vi "Filter Traces.vi"(8 "error in (no error)":errorcluster, 9 "Median Filter?":bool, 10 "Array":cluster{timestamp[], dbl[]}[](array[cluster]), 11 "Database Viewer in":refnum<class "Database Viewer.lvclass">) -> (0 "error out":errorcluster, 2 "Database Trace out":T1(array[cluster]), 3 "Database Viewer out":refnum<class "Database Viewer.lvclass">)   [LabVIEW 2019, in "Database Viewer.lvclass"]
uses:
  Database Viewer.lvclass
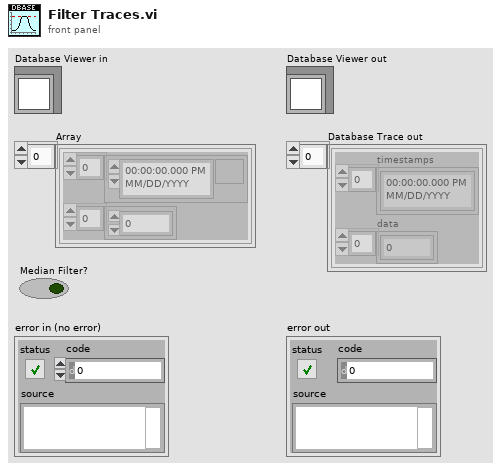
[diagram p1: front panel]
types:
  T1 = cluster{"timestamps":timestamp[], "data":dbl[]}[]
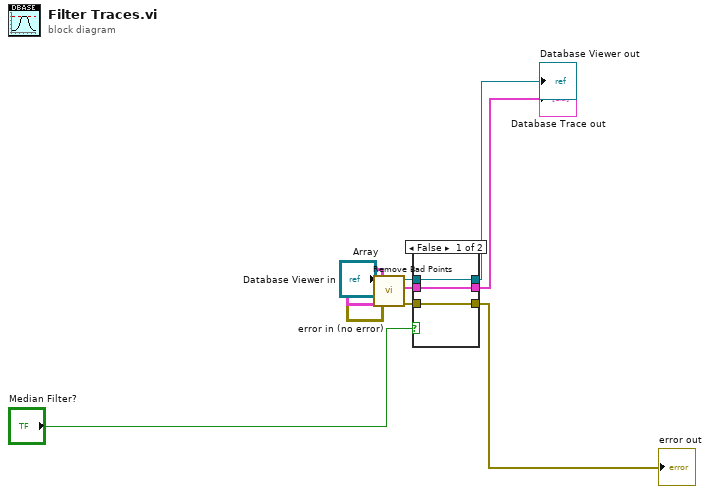
[diagram p0: block diagram]
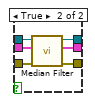
[diagram p2: hidden frame]
diagram:
  n1 = call "Remove Bad Points.vi"("error in (no error)"="error in (no error)", "Database Trace In"="Array", "Database Viewer"="Database Viewer in") -> ("error out"=w2:errorcluster, "Database Trace Out"=w7:T1, "Database Viewer out"=w9:refnum<class "Database Viewer.lvclass">)  [unwired: 6 in]
  n2 = case shown="False" "Median Filter?" {
    tunnel: w7 -> [w12 w17]
    tunnel: w2 -> [w13 w19]
    tunnel: [w12 w16] -> w5
    tunnel: [w13 w18] -> w4
    tunnel: w9 -> [w11 w15]
    tunnel: [w11 w14] -> w10
    frame False {
    }
    frame True {
      n3 = call "Median Filter.vi"("error in (no error)"=w19, "Database Trace"=w17, "Database Viewer"=w15) -> ("error out"=w18:errorcluster, "Database Trace out"=w16:T1, "Database Viewer out"=w14:refnum<class "Database Viewer.lvclass">)  [unwired: 6 in]
    }
  }
  "Database Viewer out" <- w10
  "Database Trace out" <- w5
  "error out" <- w4
